vi "UpdateBfield.vi"(5 "Force upodate (F)":bool, 7 "B [T] in":dbl, 8 "error in (no error)":errorcluster, 11 "MagSpec_Bella in":refnum<class "MagSpec_Bella.lvclass">) -> (0 "error out":errorcluster, 3 "MagSpec_Bella out":refnum<class "MagSpec_Bella.lvclass">)   [LabVIEW 2013, in "MagSpec_Bella.lvclass"]
uses:
  MagSpec_Bella.lvclass
panel:
  in  "deadband":dbl=0.05 format="%#_13g"
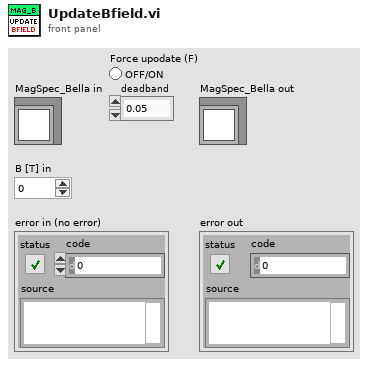
[diagram p1: front panel]
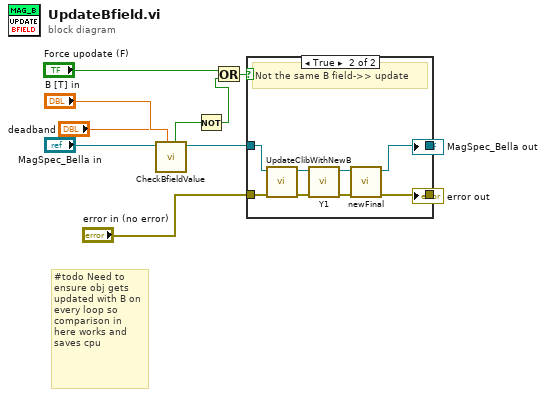
[diagram p0: block diagram]
diagram:
  # "#todo Need to ensure obj gets updated with B on every loop so comparison in here works and saves cpu"
  n1 = call "CheckBfieldValue .vi"("deadband"="deadband", "B [T] new"="B [T] in", "MagSpec_Bella in"="MagSpec_Bella in") -> ("MagSpec_Bella out"=w7:refnum<class "MagSpec_Bella.lvclass">, "Same?"=w5:bool)  [unwired: 7 in]
  n2 = Not(x=w5) -> (.not. x?=w4:bool)
  n3 = Or(x="Force upodate (F)", y=w4) -> (x .or. y?=w2:bool)
  n4 = case shown="True" w2 {
    tunnel: [w12 w21] -> w11
    tunnel: [w13 w20] -> w10
    tunnel: "error in (no error)" -> [w13 w19]
    tunnel: w7 -> [w12 w18]
    frame False {
    }
    frame True {
      # "Not the same B field->> update"
      n5 = call "UpdateClibWithNewB.vi"("error in (no error)"=w19, "MagSpec_Bella in"=w18) -> ("error out"=w15:errorcluster, "MagSpec_Bella out"=w14:refnum<class "MagSpec_Bella.lvclass">)  [unwired: 8 in]
      n6 = call "Y1.vi"("error in (no error)"=w15, "MagSpec_Bella in"=w14) -> ("error out"=w16:errorcluster, "MagSpec_Bella out"=w17:refnum<class "MagSpec_Bella.lvclass">)  [unwired: 8 in]
      n7 = call "newFinal.vi"("error in (no error)"=w16, "MagSpec_Bella in"=w17) -> ("error out"=w20:errorcluster, "MagSpec_Bella out"=w21:refnum<class "MagSpec_Bella.lvclass">)  [unwired: 8 in]
    }
  }
  "MagSpec_Bella out" <- w11
  "error out" <- w10
